vi "run.update_endtime.request.vi"(8 "error in (no error)":errorcluster, 9 "End":timestamp format="%<%x %.3X>T", 10 "Run":refnum<class "Run.lvclass">) -> (0 "error out":errorcluster, 2 "Request Body":string)   [LabVIEW 2020, in "Nominal Client.lvclass"]
uses:
  Nominal Client.lvclass
  Run/Run.lvclass
  Run/Run.lvclass/Run.ctl
  39a8f659-5d8a-46da-a3aa-f8275ef01e22.vi
  dbbb6b07-2306-4fbf-be02-61899f0ec727.vi
  ecb75084-90d7-4e08-bee6-04057d0c25d0.vi
  Run/assets.get.vi
  Run/assets.get.vi/fc990382-c15b-405e-8523-435b97eca7cf.vi
  Run/assets.get.vi/fc990382-c15b-405e-8523-435b97eca7cf.vi/32c3acc2-0975-485a-8283-62feb0f3dc4f.vi
  Run/run_properties.get.vi
  <vilib>/LabVIEW Open Source Project/Epoch Date & Time/epoch.UNIX/Epoch.UNIX.lvclass
  C:/Program Files/National Instruments/LabVIEW 2020/vi.lib/LabVIEW Open Source Project/Epoch Date & Time/epoch/Epoch.lvclass
  <vilib>/LabVIEW Open Source Project/Epoch Date & Time/Get Epoch Time.vi
  Run/update.cache.vi
  <vilib>/JDP Science/JSONtext/JSON text to Variant.vi
  <vilib>/JDP Science/JSONtext/Variant to JSON Text.vi
  <vilib>/JDP Science/JSONtext/support/Format JSON Object.vi
  <vilib>/JDP Science/JSONtext/LVClass Serializer/JSONtext LVClass Serializer.lvclass
  Nominal Client.lvclass/Nominal Client.ctl
  <vilib>/JDP Science/JSONtext/JSONtext.lvlib
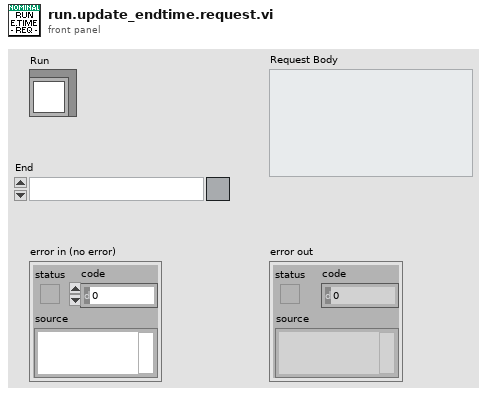
[diagram p1: front panel]
types:
  T1 = cluster{"secondsSinceEpoch":i64, "offsetNanoseconds":i64}
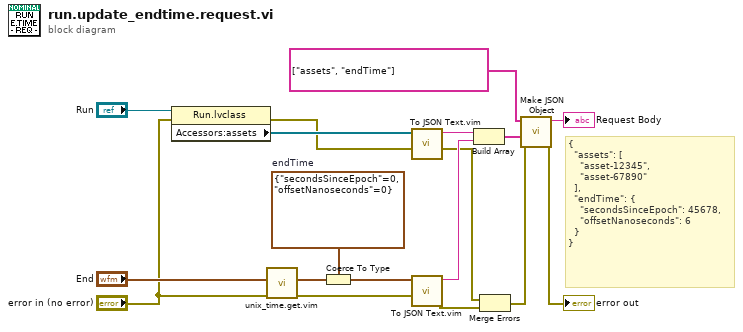
[diagram p0: block diagram]
diagram:
  w11 = T1 {"secondsSinceEpoch"=0, "offsetNanoseconds"=0}  # endTime
  # "{\n  \"assets\": [\n    \"asset-12345\",\n    \"asset-67890\"\n  ],\n  \"endTime\": {\n    \"secondsSinceEpoch\": 45678,\n    \"offsetNanoseconds\": 6\n  }\n}"
  n1 = property class="Run.lvclass"(reference="Run", error in="error in (no error)") -> (error out=w9:errorcluster, "Accessors:assets"=w15:refnum<class "asset.lvclass">[])  [unwired: 1 out]
  n2 = call "unix_time.get.vim"("Time Stamp (empty: now) [single or array]"="End") -> ("UNIX Timestamp"=w14:cluster{"Seconds":i64, "Nanoseconds":i64})  [unwired: 10 in]
  n3 = Coerce To Type(0:w14, 1:w11) -> (2:w10:T1)
  n4 = call "To JSON Text.vim"("error in (no error)"=w9, "Anything"=w15) -> ("error out"=w6:errorcluster, "<JSON>"=w12:string)  [unwired: 8 in]
  n5 = call "To JSON Text.vim"("error in (no error)"="error in (no error)", "Anything"=w10) -> ("error out"=w5:errorcluster, "<JSON>"=w7:string)  [unwired: 8 in]
  n6 = Build Array(w12, w7) -> (w3:string[])
  n7 = Merge Errors(w6, w5) -> (w4:errorcluster)
  n8 = call <vilib>:"Make JSON Object.vi"("error in (no error)"=w4, "JSON Items"=w3, "Item Names"=string[] ["assets", "endTime"]) -> ("error out"=→"error out":errorcluster, "<JSON>"=→"Request Body":string)  [unwired: 7 in]
